vi "Init.vi"(8 "error in (no error)":errorcluster, 11 "UI Actor in":refnum<class "UI Actor.lvclass">) -> (0 "error out":errorcluster, 3 "UI Actor out":refnum<class "UI Actor.lvclass">)   [LabVIEW 2020, in "UI Actor.lvlib" / "UI Actor.lvclass"]
uses:
  UI Actor.lvclass
  UI Actor.lvclass/UI Actor.ctl
  Implementations/NXP/NXP.lvclass
  D:/Fork/IVProyecto_3P/Abstract/Serial Device/Serial Device.lvclass
  Implementations/Simulado/Simulado.lvclass
  Abstract/Serial Device/Serial Device.lvclass
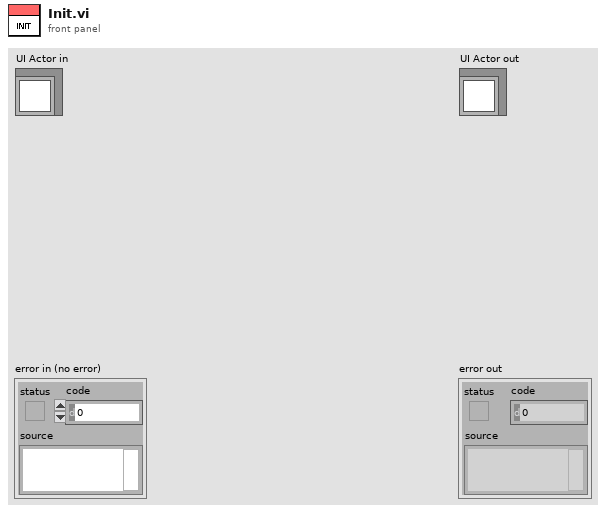
[diagram p1: front panel]
types:
  T1 = typedef "Control 1.ctl" = string
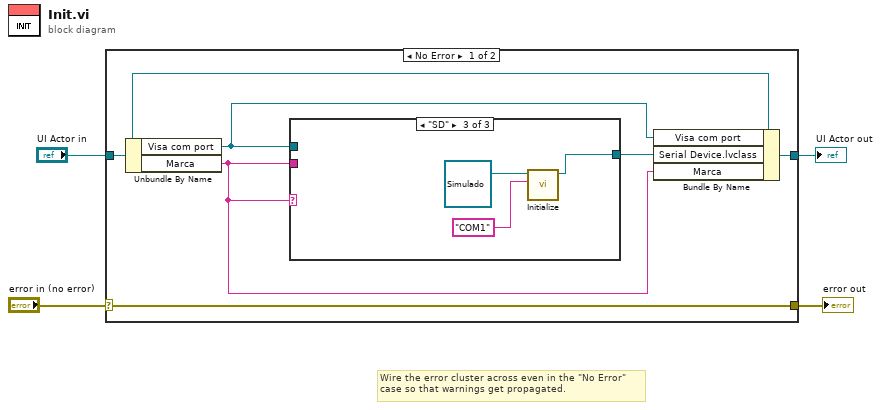
[diagram p0: block diagram]
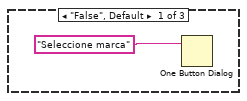
[diagram p2: hidden frame]
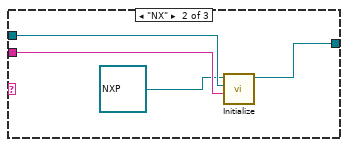
[diagram p3: hidden frame]
diagram:
  # "Wire the error cluster across even in the \"No Error\"\ncase so that warnings get propagated."
  n1 = case shown="No Error" "error in (no error)" {
    selector: "error in (no error)" -> [w10 w20]
    tunnel: [w10 w20] -> w3
    tunnel: [w8 w19] -> w1
    tunnel: "UI Actor in" -> [w9 w19]
    frame No Error {
      n2 = Unbundle By Name(w9) -> ("Visa com port"=w6:refnum<visa-resource-name>, "Marca"=w5:T1)
      n3 = case shown="\"SD\"" w5 {
        tunnel: w6 -> [_ w13 _]
        tunnel: w5 -> [_ w15 _]
        tunnel: [_ w14 w18] -> w7
        frame "False", Default {
          n4 = One Button Dialog(message="Seleccione marca") -> ()  [unwired: 1 in, 1 out]
        }
        frame "NX" {
          n5 = call-dynamic "Initialize.vi"("Marca"=w15, "Puerto Com"=w13, "object in"=refnum<class "NXP.lvclass"> refnum ("NXP.lvclass")) -> ("object out"=w14:refnum<class "NXP.lvclass">)  [unwired: 7 in, 1 out]
        }
        frame "SD" {
          n6 = call-dynamic "Initialize.vi"("Puerto Com"="COM1", "object in"=refnum<class "Simulado.lvclass"> refnum ("Simulado.lvclass")) -> ("object out"=w18:refnum<class "Simulado.lvclass">)  [unwired: 8 in, 1 out]
        }
      }
      n7 = Bundle By Name(cluster=w9, "Visa com port"=w6, "Serial Device.lvclass"=w7, "Marca"=w5) -> (w8:refnum<class "UI Actor.lvclass">)
    }
    frame Error {
    }
  }
  "error out" <- w3
  "UI Actor out" <- w1
